vi "Find Average Center_01282025.vi"(5 "Position":i32, 7 "Tray Number":i32, 8 "Assembly Type":string, 9 "XYZTheta":dbl[](array[numeric]), 11 "Gantry In":refnum<k24>) -> (1 "XYZTheta":dbl[](array[numeric]) format="%.6g", 3 "Gantry Out":refnum<k24>)   [LabVIEW 2021, in "Component Tray.lvclass"]
uses:
  Component Tray.lvclass
  Find Component.ctl
  Controller/Camera/Machine Vision.ctl
  C:/Program Files (x86)/Aerotech/A3200/LabVIEW/2010/Bin/Aerotech.A3200.dll
  Program Files (x86)/Aerotech/A3200/LabVIEW/2010/Bin/Aerotech.A3200.dll
  Controller/Camera/Image processing.ctl
  Controller/Camera/Camera settings.ctl
  Controller/Camera/Material.ctl
  Controller/Camera/Edmund Optics/Edmund Optics.lvclass
  C:/Users/User/Documents/Jessica_Code/Jessica_code_08062024/Gantry-CMU/UCSB-Gantry-HEP-main/Classes/Controller/Camera/Camera.lvclass
  Controller/Camera/Camera.lvclass
  Controller/Motion/A3200/A3200.lvclass
  Controller/Motion/Motion.lvclass
  Routine/TypeOfHexaboard.ctl
  Routine/Routine.lvclass
panel:
  out "Low Speed":bool
  out "X":bool
  out "Y":bool
  out "Z":bool
  out "High Speed":bool
  in  "Go to Top Right":bool
  in  "Go to Bottom Right":bool
  out "Program Stopped":bool
  out "XY Graph":cluster{"X":dbl, "Y":dbl}[](graph)
  out "Sensor ID Location":dbl[](array[numeric])
  in  "Go to Sensor ID":bool
  out "CH1 Location":dbl[](array[numeric])
  in  "Verify CH1":bool
  out "CH1 correct?":bool
  in  "Go to CH1":bool
  in  "Focus step size":dbl format="%#_13g"
  in  "number of focus steps":i32
  out "Average Strength":dbl
  in  "Focus":bool
  in  "Material":T1
  out "All fiducials recorded":bool
  in  "Override presets":bool
  in  "Camera settings":T2={"Gamma"=1.6, "Gain"=0, "Sharpness"=0, "Contrast"=0.0, "Exposure"=0.0078125} {"Exposure" min=0.000244140625 max=0.5 scale=0.0002..0.5; "Contrast" min=0.0 max=1.0 scale=0.001..1.0; "Sharpness" min=0 max=2 step=1 scale=0.0..2.0; "Gain" min=0 max=100 step=1 scale=0.1..100.0; "Gamma" min=0.01 max=10.0 scale=0.01..10.0}
  in  "Image processing":T3={"Brightness"=128.0, "Contrast"=45.0, "Gamma"=1.0471123} {"Brightness" scale=0.0..400.0; "Contrast" scale=0.0..90.0; "Gamma" scale=0.005..5.0}
  in  "Machine Vision":T4=enum."Sensor Fiducials"
  out "Gantry":dbl[](array[numeric]) format="%.6g"
  out "Sum":dbl[](array[numeric]) format="%.6g"
  out "Bottom Right XY":dbl[](array[numeric]) format="%.6g"
  out "Bottom Left XY":dbl[](array[numeric]) format="%.6g"
  out "Top Right XY":dbl[](array[numeric]) format="%.6g"
  out "Top Left XY":dbl[](array[numeric]) format="%.6g"
  in  "Record Bottom Left":bool
  in  "Record Bottom Right":bool
  in  "Record Top Right":bool
  in  "Record Top Left":bool
  in  "Go to Bottom Left":bool
  in  "Go to Top Left":bool
  in  "Joystick":bool
  out "Camera":dbl[](array[numeric]) format="%.6g"
  in  "Go to Center":bool
  in  "Component":T5
  in  "Stop Program":bool
  out "Image":T6(plugin-control)
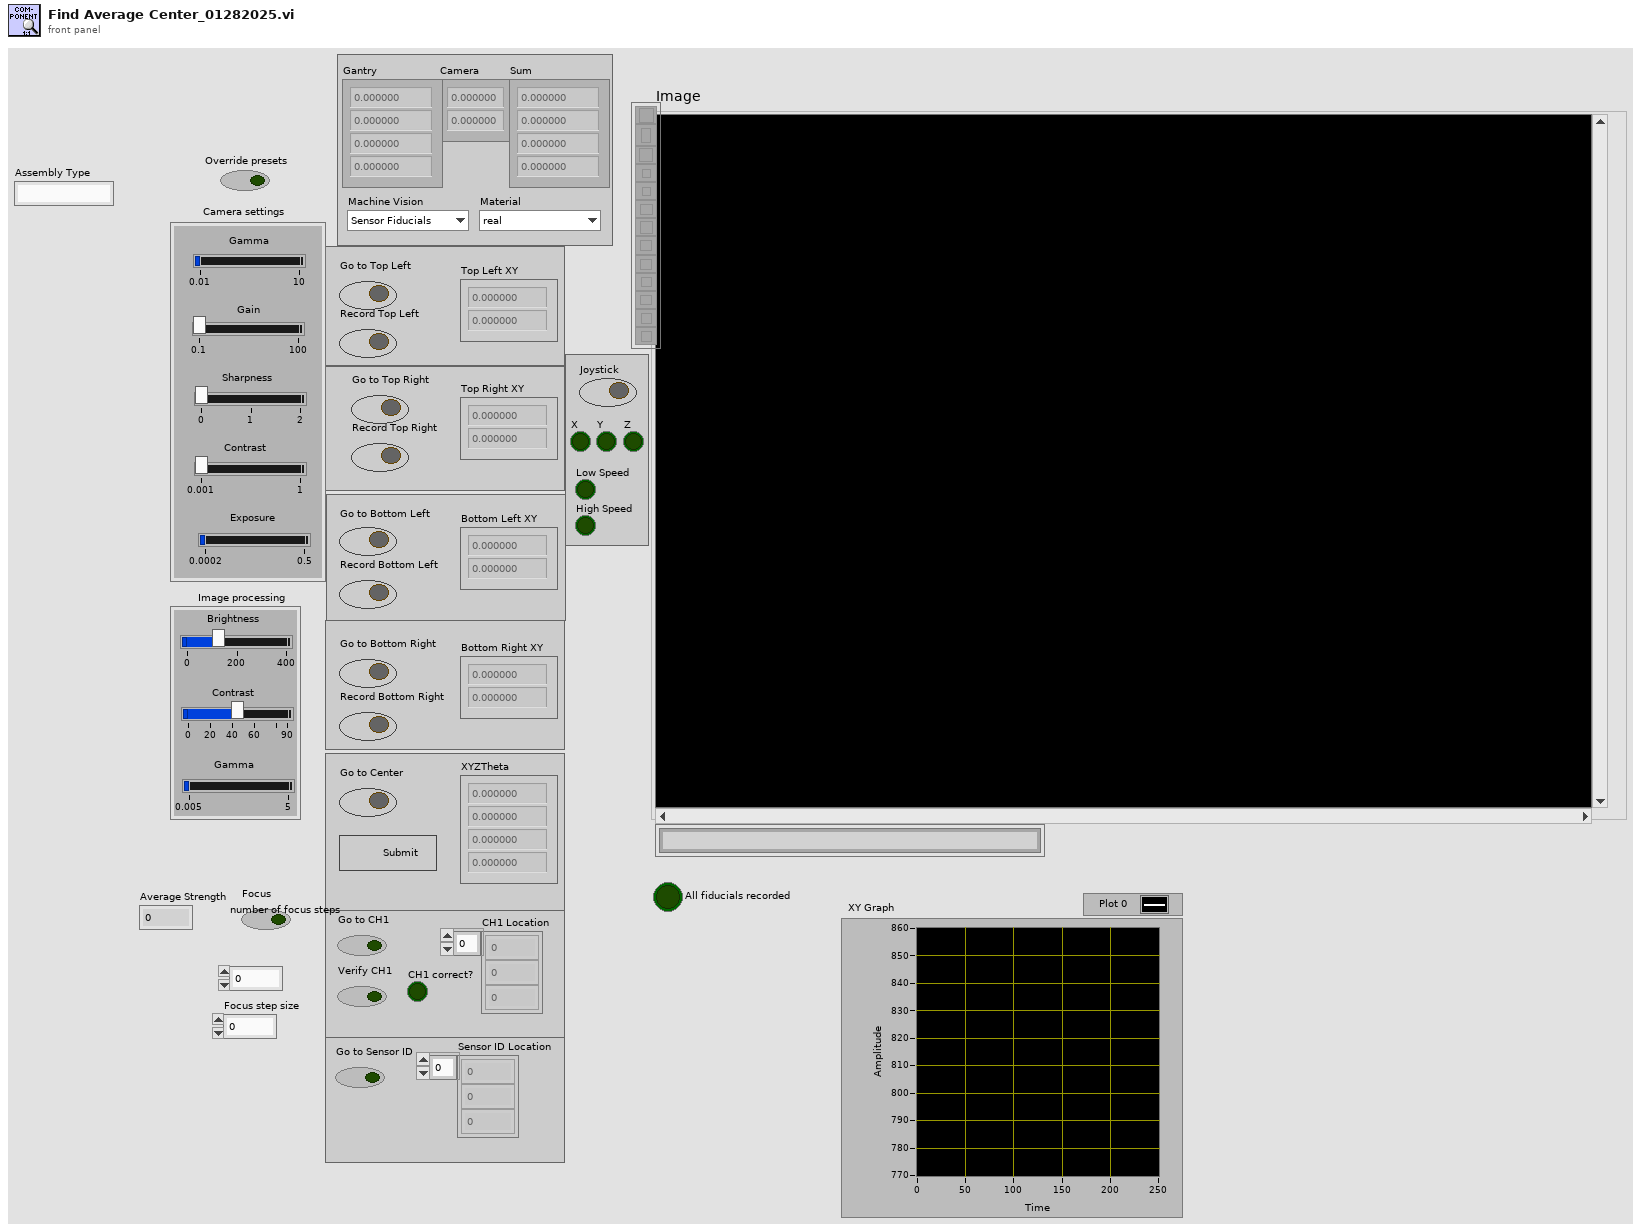
[diagram p1: front panel]
types:
  T1 = typedef "Camera.lvclass/Material.ctl" = enum16{"real", "dummy", "PETG"}
  T2 = typedef "Camera.lvclass/Camera settings.ctl" = cluster{"Gamma":dbl, "Gain":i64, "Sharpness":i64, "Contrast":dbl, "Exposure":dbl}
  T3 = typedef "Camera.lvclass/Image processing.ctl" = cluster{"Brightness":sgl, "Contrast":sgl, "Gamma":sgl}
  T4 = typedef "Camera.lvclass/Machine Vision.ctl" = enum16{"None", "Tray Fiducials", "V3 Sensor Circle", "Partial Hexaboard", "HPK Silicon", "Partial Hexaboard Test", "100um dot", "Hexaboard", "Corner (TL, BR)", "Corner (BL, TR)", "V3 Sensor Cross", "test", "Sensor Fiducials"}
  T5 = typedef "Component Tray.lvclass/Find Component.ctl" = cluster{"New Fiducials":dbl[], "Past Fiducials":dbl[], "XYZTheta":dbl[], "Fiducials Path":path, "Position":i32, "CH1 Location":dbl[], "Sensor ID Location":dbl[]}
  T6 = typedef "IMAQ Image.ctl" = refnum<image>
  T7 = typedef "Routine.lvclass/TypeOfHexaboard.ctl" = enum16{"Full Sensor", "Full PCB", "Right Partial PCB", "Right Partial Sensor", "Al Dummy Right Partial Sensor"}
  T8 = typedef "File Paths.ctl" = cluster{"Glue Pattern Folder":path, "Carrier Tray Folder":path, "Pick Up Tool Fixture Folder":path, "Components Folder":path, "Bellows Tool Offset.txt":path, "Pick Up Tool Offset.txt":path, "Dispense Tip Offset.txt":path, "Log Files":path, "Gantry Assembly Map.txt":path, "Syringe and offset map.txt":path, "Controllers Folder":path, "Local dbase config":path}
  T9 = enum8{"Enabled", "Disabled", "Disabled and Grayed Out"}
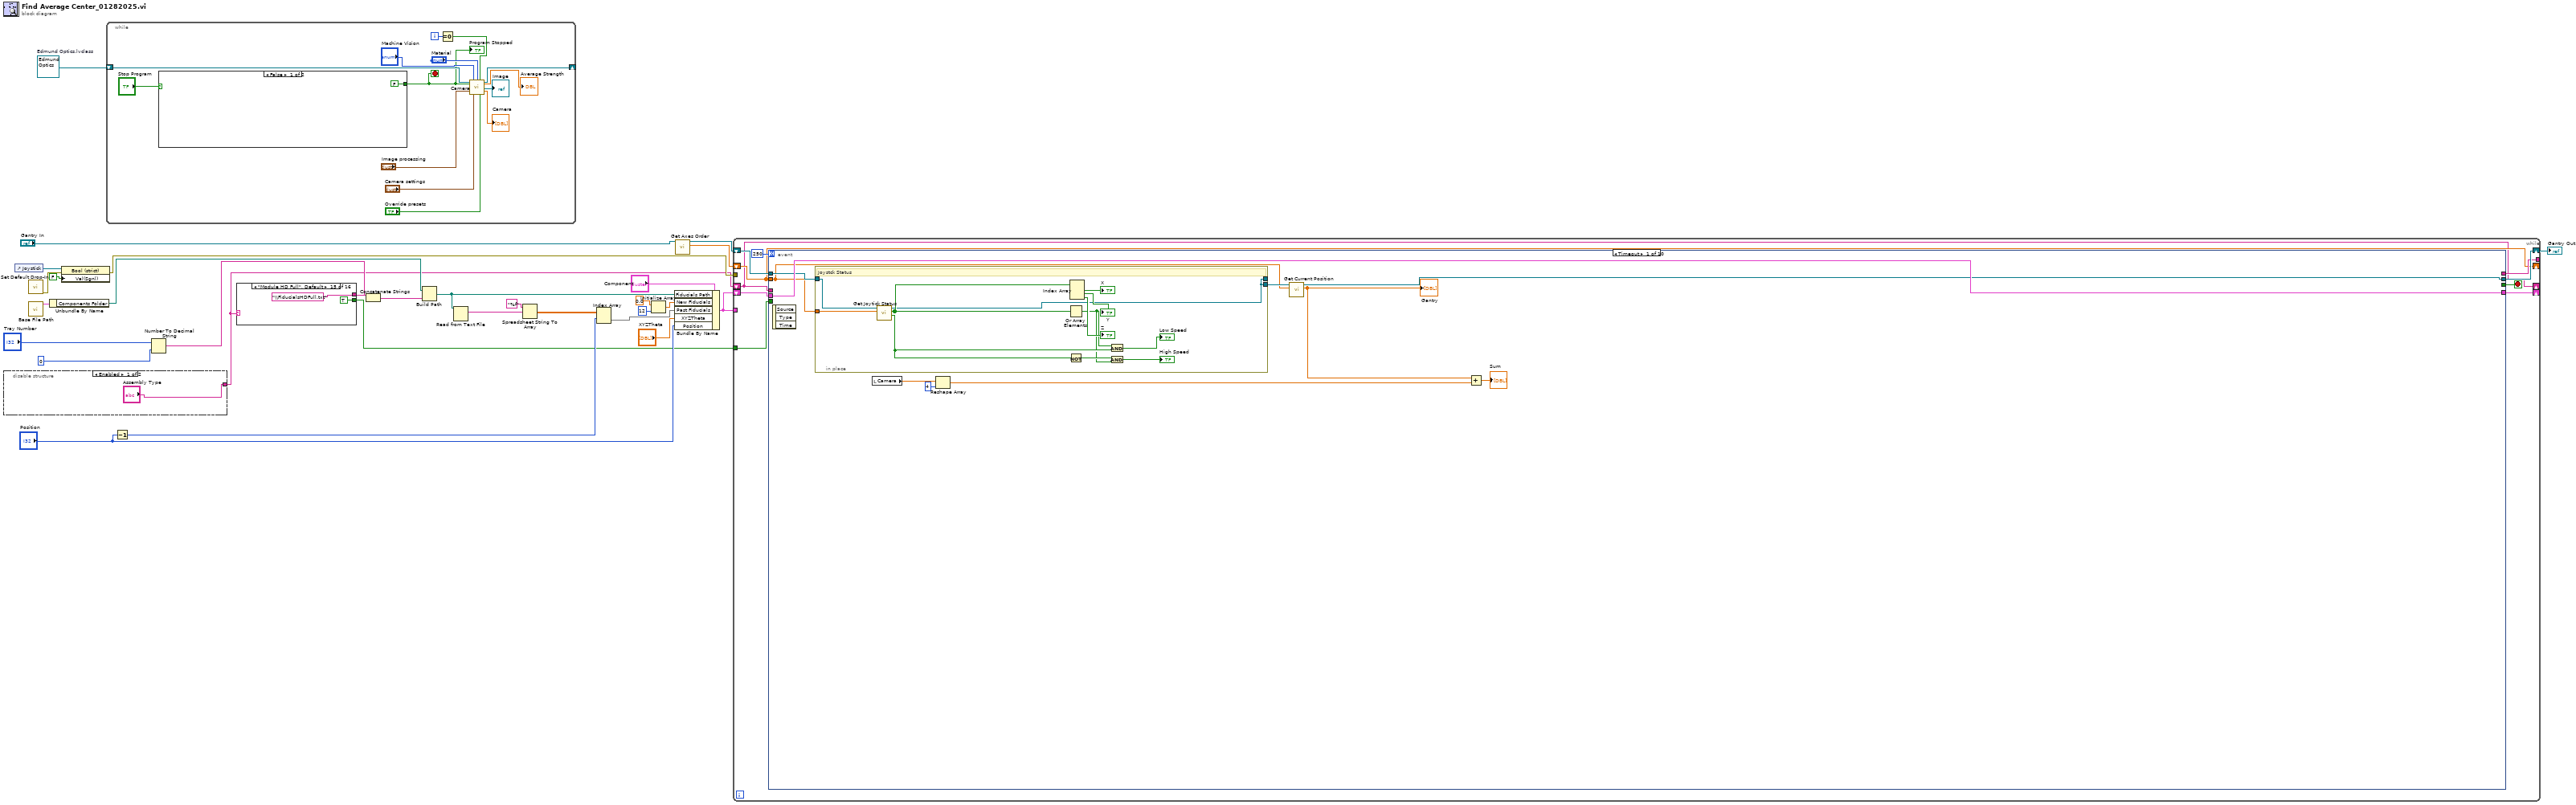
[diagram p0: block diagram]
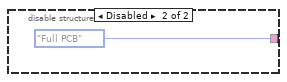
[diagram p2: hidden frame]
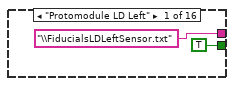
[diagram p3: hidden frame]
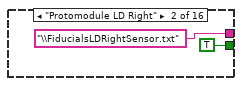
[diagram p4: hidden frame]
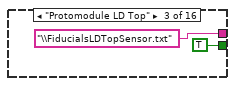
[diagram p5: hidden frame]
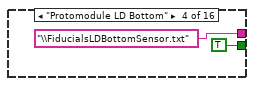
[diagram p6: hidden frame]
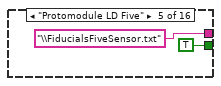
[diagram p7: hidden frame]
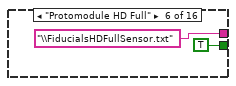
[diagram p8: hidden frame]
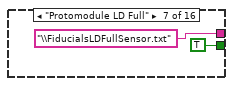
[diagram p9: hidden frame]
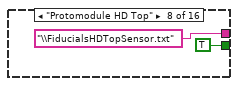
[diagram p10: hidden frame]
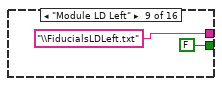
[diagram p11: hidden frame]
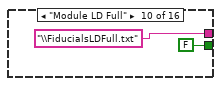
[diagram p12: hidden frame]
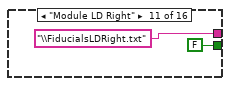
[diagram p13: hidden frame]
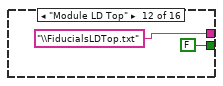
[diagram p14: hidden frame]
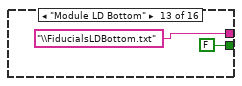
[diagram p15: hidden frame]
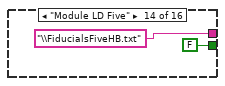
[diagram p16: hidden frame]
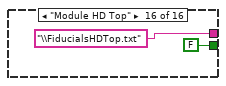
[diagram p17: hidden frame]
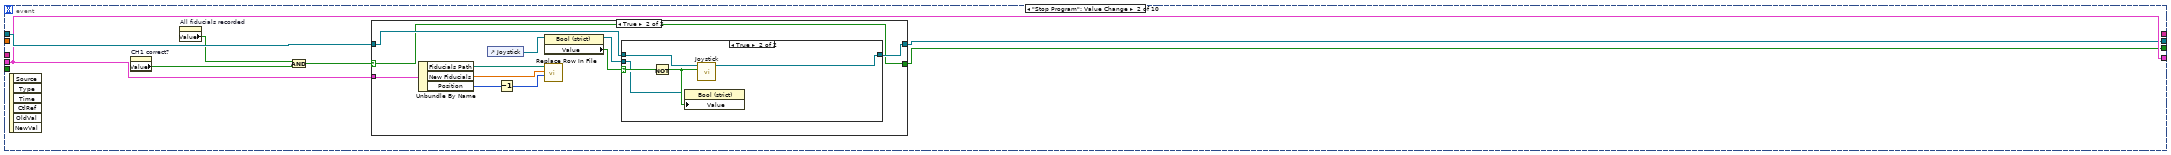
[diagram p18: hidden frame]
diagram:
  w27 = refnum<class "Edmund Optics.lvclass"> refnum  # Edmund Optics.lvclass
  n1 = disable-structure shown="Enabled" {
    disable-tunnel: ["Assembly Type" TypeOfHexaboard."Full PCB" ("Type of Hexaboard")] -> w1
    frame Enabled {
    }
    frame Disabled {
    }
  }
  n2 = control-ref of="Joystick"() -> (w30:refnum<vi>)
  n3 = call "Set Default Drop-In.vi"() -> ("error out"=w8:errorcluster)  [unwired: 11 in]
  n4 = call "Base File Path.vi"() -> ("Paths Out"=w18:T8)  [unwired: 11 in]
  n5 = Unbundle By Name(w18) -> ("Components Folder"=w20:path)
  n6 = property class="Bool (strict)"(reference=w30, error in=w8, "Val(Sgnl)"=FALSE) -> (error out=w28:errorcluster)  [unwired: 1 out]
  n7 = while {
    shift-right: [w43] -> _
    shift-left: w27 -> [w47]
    i -> [w39]
    stop <- w34 stop-if-true
    n8 = case shown="False" "Stop Program" {
      tunnel: [FALSE w49] -> w34
      frame False {
      }
      frame True {
        n9 = property on="All fiducials recorded" class="Bool (strict)"() -> ("Value"=w52:bool)  [unwired: 2 in, 2 out]
        n10 = property on="CH1 correct?" class="Bool (strict)"() -> ("Value"=w50:bool)  [unwired: 2 in, 2 out]
        n11 = And(x=w52, y=w50) -> (x .and. y?=w51:bool)
        n12 = case shown="False" w51 {
          tunnel: [FALSE TRUE] -> w49
          frame False {
            n13 = One Button Dialog(message="At least one fiducial not recorded or component orientation not verified.") -> ()  [unwired: 1 in, 1 out]
          }
          frame True {
            n14 = property on="All fiducials recorded" class="Bool (strict)"("Val(Sgnl)"=FALSE) -> ()  [unwired: 2 in, 2 out]
          }
        }
      }
    }
    "Program Stopped" <- w34
    n15 = Equal To 0?(x=w39) -> (x = 0?=w38:bool)
    n16 = call "Camera.vi"("Camera in"=w47, "Stop"=w34, "BCG Image Processing"="Image processing", "Machine Vision"="Machine Vision", "Camera settings"="Camera settings", "Material"="Material", "Loop 0"=w38, "Override presets"="Override presets") -> ("Camera out"=w43:refnum<class "Edmund Optics.lvclass">, "Average Strength"=→"Average Strength":dbl, "Image"=→"Image":T6, "Camera"=→"Camera":dbl[])  [unwired: 5 in, 3 out]
  }
  n17 = Decrement(x="Position") -> (x-1=w9:i32)
  n18 = Number To Decimal String(number="Tray Number", width (-)=i16 0) -> (decimal integer string=w21:string)
  n19 = case shown="\"Module HD Full\", Default" w1 {
    tunnel: ["\\FiducialsLDLeftSensor.txt" ("string") "\\FiducialsLDRightSensor.txt" ("string") "\\FiducialsLDTopSensor.txt" ("string") "\\FiducialsLDBottomSensor.txt" ("string") "\\FiducialsFiveSensor.txt" ("string") "\\FiducialsHDFullSensor.txt" ("string") "\\FiducialsLDFullSensor.txt" ("string") "\\FiducialsHDTopSensor.txt" ("string") "\\FiducialsLDLeft.txt" ("string") "\\FiducialsLDFull.txt" ("string") "\\FiducialsLDRight.txt" ("string") "\\FiducialsLDTop.txt" ("string") "\\FiducialsLDBottom.txt" ("string") "\\FiducialsFiveHB.txt" ("string") "\\FiducialsHDFull.txt" ("string") "\\FiducialsHDTop.txt" ("string")] -> w22
    tunnel: [TRUE TRUE TRUE TRUE TRUE TRUE TRUE TRUE FALSE FALSE FALSE FALSE FALSE FALSE TRUE FALSE] -> w5
    frame "Protomodule LD Left" {
    }
    frame "Protomodule LD Right" {
    }
    frame "Protomodule LD Top" {
    }
    frame "Protomodule LD Bottom" {
    }
    frame "Protomodule LD Five" {
    }
    frame "Protomodule HD Full" {
    }
    frame "Protomodule LD Full" {
    }
    frame "Protomodule HD Top" {
    }
    frame "Module LD Left" {
    }
    frame "Module LD Full" {
    }
    frame "Module LD Right" {
    }
    frame "Module LD Top" {
    }
    frame "Module LD Bottom" {
    }
    frame "Module LD Five" {
    }
    frame "Module HD Full", Default {
    }
    frame "Module HD Top" {
    }
  }
  n20 = Concatenate Strings "Concatenate Strings"(w21, w22) -> (w23:string)
  n21 = Build Path(base path=w20, name or relative path=w23) -> (appended path=w12:path)
  n22 = Read from Text File(file (use dialog)=w12) -> (text=w24:string)  [unwired: 3 in, 3 out]
  n23 = Spreadsheet String To Array(format string="%f", spreadsheet string=w24) -> (array=w26:dbl[][])  [unwired: 2 in]
  n24 = Index Array "Index Array"(array=w26, index (row)=w9) -> (element=w16:dbl[])  [unwired: 1 in]
  n25 = Initialize Array(0.0 ("element"), 12 ("dimension size")) -> (w15:dbl[])
  n26 = Bundle By Name "Bundle By Name"(cluster="Component", "Fiducials Path"=w12, "New Fiducials"=w15, "Past Fiducials"=w16, "XYZTheta"="XYZTheta", "Position"="Position") -> (w6:T5)
  n27 = call "Get Axes Order.vi"("Gantry In"="Gantry In") -> ("Axes Order"=w2:dbl[], "Gantry Out"=w3:refnum<k24>)  [unwired: 8 in, 1 out]
  n28 = while {
    shift-right: [w96] -> _
    shift-left: w6 -> [w97]
    tunnel: w28 -> [_]
    shift-right: [w93] -> w7
    shift-left: w3 -> [w94]
    tunnel: w6 -> [_]
    tunnel: [w92] -> _
    tunnel: w5 -> [w91]
    shift-right: [w90] -> _
    shift-left: w2 -> [w90]
    shift-right: [w89] -> _
    shift-left: w1 -> [w89]
    stop <- w98 stop-if-true
    n29 = event shown="[0] Timeout" {
      selector: _ -> [_ _ _ _ _ _ _ _ _ _]
      dyn-events: _ -> [_ _ _ _ _ _ _ _ _ _]
      timeout: 250 -> [_ _ _ _ _ _ _ _ _ _]
      tunnel: [_ w124 _ _ _ _ _ _ _ _] -> w98
      tunnel: w97 -> [w107 w126 w163 w227 w366 w414 w421 w436 w451 w461]
      tunnel: [w107 w126 w163 w226 w366 w414 w421 w436 w451 w461] -> w96
      tunnel: w94 -> [w101 w127 w162 w218 w368 w413 w417 w432 w447 w462]
      tunnel: [w103 w125 w159 w216 w367 w411 w415 w430 w445 w462] -> w93
      tunnel: w89 -> [_ _ w156 w215 _ _ _ _ _ _]
      tunnel: [_ _ w156 _ _ _ _ _ _ _] -> w92
      tunnel: w91 -> [_ _ w147 w191 _ _ _ _ _ _]
      tunnel: w90 -> [w99 _ _ w190 w356 _ _ _ _ _]
      event Timeout {
        n30 = event-data() -> ()  [unwired: 1 in, 3 out]
        n31 = in-place {
          in-place-border: w101 -> [w120]
          in-place-border: [w109] -> _
          in-place-border: w99 -> [w119]
          in-place-border: [w109] -> w100
          # "Joystck Status"
          n32 = call "Get Joytick Status.vi"("Axes Order"=w119, "Gantry In"=w120) -> ("JoystickLowSpeedActive"=w113:bool, "Joystick Status"=w115:bool[], "Gantry Out"=w109:refnum<k24>)  [unwired: 6 in, 1 out]
          n33 = Or Array Elements(Boolean array=w115) -> (logical OR=w111:bool)
          n34 = Not(x=w113) -> (.not. x?=w112:bool)
          n35 = Index Array(array=w115) -> (element #1=→"X":bool, element #2=→"Y":bool, element #3=→"Z":bool)  [unwired: 3 in]
          n36 = And(x=w111, y=w113) -> (x .and. y?=→"Low Speed":bool)
          n37 = And(x=w112, y=w111) -> (x .and. y?=→"High Speed":bool)
        }
        n38 = local read "Camera"() -> (w106:dbl[])
        n39 = Reshape Array(w106, 4 ("dimension size")) -> (w104:dbl[])
        n40 = call "Get Current Position.vi"("Axes Order"=w99, "Gantry In"=w100) -> ("XYZTheta Out"=w102:dbl[], "Gantry Out"=w103:refnum<k24>)  [unwired: 7 in, 1 out]
        "Gantry" <- w102
        n41 = Add(x=w102, y=w104) -> (x+y=→"Sum":dbl[])
      }
      event "Stop Program": Value Change {
        n42 = event-data() -> ()  [unwired: 1 in, 6 out]
        n43 = property on="CH1 correct?" class="Bool (strict)"() -> ("Value"=w123:bool)  [unwired: 2 in, 2 out]
        n44 = property on="All fiducials recorded" class="Bool (strict)"() -> ("Value"=w122:bool)  [unwired: 2 in, 2 out]
        n45 = And(x=w122, y=w123) -> (x .and. y?=w121:bool)
        n46 = case shown="True" w121 {
          selector: w121 -> [w128 w137]
          tunnel: w127 -> [w129 w139]
          tunnel: w126 -> [_ w140]
          tunnel: [w129 w138] -> w125
          tunnel: [w128 w137] -> w124
          frame False {
          }
          frame True {
            n47 = Unbundle By Name(w140) -> ("Fiducials Path"=w134:path, "New Fiducials"=w133:dbl[], "Position"=w135:i32)
            n48 = control-ref of="Joystick"() -> (w131:refnum<vi>)
            n49 = Decrement(x=w135) -> (x-1=w136:i32)
            n50 = property class="Bool (strict)"(reference=w131) -> (reference out=w130:refnum<vi>, "Value"=w132:bool)  [unwired: 1 in, 1 out]
            n51 = call "Replace Row In File.vi"("Index"=w136, "Insert Array"=w133, "Path"=w134) -> ()  [unwired: 8 in, 1 out]
            n52 = case shown="True" w132 {
              selector: w132 -> [_ w146]
              tunnel: w139 -> [w141 w145]
              tunnel: [w141 w144] -> w138
              tunnel: w130 -> [_ w142]
              frame False {
              }
              frame True {
                n53 = Not(x=w146) -> (.not. x?=w143:bool)
                n54 = property class="Bool (strict)"(reference=w142, "Value"=w143) -> ()  [unwired: 1 in, 2 out]
                n55 = call "Joystick.vi"("Joystick"=w143, "Gantry In"=w145) -> ("Gantry Out"=w144:refnum<k24>)  [unwired: 8 in, 1 out]
              }
            }
          }
        }
      }
      event "Go to Top Left", "Go to Bottom Left", "Go to Bottom Right", "Go to Top Right": Value Change {
        n56 = event-data() -> ()  [unwired: 1 in, 6 out]
        n57 = disable-structure shown="Enabled" {
          disable-tunnel: w162 -> [w169 _]
          disable-tunnel: [w168 _] -> w161
          frame Enabled {
            n58 = control-ref of="Joystick"() -> (w167:refnum<vi>)
            n59 = property class="Bool (strict)"(reference=w167) -> (reference out=w170:refnum<vi>, "Value"=w171:bool)  [unwired: 1 in, 1 out]
            n60 = case shown="True" w171 {
              selector: w171 -> [_ w177]
              tunnel: w169 -> [w172 w175]
              tunnel: [w172 w173] -> w168
              tunnel: w170 -> [_ w176]
              frame False {
              }
              frame True {
                n61 = Not(x=w177) -> (.not. x?=w174:bool)
                n62 = call "Joystick.vi"("Joystick"=w174, "Gantry In"=w175) -> ("Gantry Out"=w173:refnum<k24>)  [unwired: 8 in, 1 out]
                n63 = property class="Bool (strict)"(reference=w176, "Value"=w174) -> ()  [unwired: 1 in, 2 out]
              }
            }
          }
          frame Disabled {
          }
        }
        n64 = Unbundle By Name(w163) -> ("Past Fiducials"=w165:dbl[])
        n65 = Build Array "Build Array"("Go to Top Left", "Go to Top Right", "Go to Bottom Left", "Go to Bottom Right") -> (w166:bool[])
        n66 = Select(t=T9."Enabled" ("Disabled"), s=w147, f=T9."Disabled and Grayed Out" ("Disabled")) -> (s? t:f=w148:T9)
        n67 = Select(t=T9."Enabled" ("Disabled"), s=w147, f=T9."Disabled and Grayed Out" ("Disabled")) -> (s? t:f=w151:T9)
        n68 = for {
          tunnel: w166 -> [w189] mode=indexing
          tunnel: w165 -> [w188]
          tunnel: [w183] -> w164 if=w189
          i -> [w186]
          n69 = Multiply(x=w186, y=3) -> (x*y=w184:i32)
          n70 = Array Subset "Array Subset"(array=w188, index=w184, length=3) -> (w183:dbl[])
        }
        n71 = property on="Go to Bottom Right" class="Bool"("DisabledEnum"=w148) -> ()  [unwired: 2 in, 2 out]
        n72 = property on="Go to Top Right" class="Bool"("DisabledEnum"=w151) -> ()  [unwired: 2 in, 2 out]
        n73 = call "ClearXYZTheta Go.vi"("XYZTheta In"=w164, "Gantry In"=w161) -> ("Gantry Out"=w160:refnum<k24>)  [unwired: 7 in, 2 out]
        n74 = flat-sequence {
          tunnel: w160 -> [w182]
          tunnel: [w179] -> w159
          frame #0 {
            w178 = TRUE
            n75 = control-ref of="Joystick"() -> (w181:refnum<vi>)
            n76 = call "Joystick.vi"("Joystick"=w178, "Gantry In"=w182) -> ("error out"=w180:errorcluster, "Gantry Out"=w179:refnum<k24>)  [unwired: 8 in]
            n77 = property on="Property Node" class="Bool (strict)"(reference=w181, error in=w180, "Value"=w178) -> ()  [unwired: 2 out]
          }
        }
      }
      event "Record Top Left", "Record Top Right", "Record Bottom Right", "Record Bottom Left": Value Change {
        n78 = event-data() -> ()  [unwired: 1 in, 1 out]
        n79 = call "Get Current Position.vi"("Axes Order"=w190, "Gantry In"=w218) -> ("XYZTheta Out"=w217:dbl[], "Gantry Out"=w216:refnum<k24>)  [unwired: 7 in, 1 out]
        n80 = control-ref of="Top Left XY"() -> (w213:refnum<vi>)
        n81 = control-ref of="Bottom Left XY"() -> (w211:refnum<vi>)
        n82 = local read "Camera"() -> (w221:dbl[])
        n83 = control-ref of="Bottom Right XY"() -> (w210:refnum<vi>)
        n84 = control-ref of="Top Right XY"() -> (w212:refnum<vi>)
        n85 = Reshape Array(w221, 3 ("dimension size")) -> (w220:dbl[])
        n86 = Build Array "Build Array"(w213, w212, w211, w210) -> (w225:refnum<vi>[])
        n87 = Add(x=w217, y=w220) -> (x+y=w219:dbl[])
        n88 = Select(t=T9."Enabled" ("Disabled"), s=w191, f=T9."Disabled and Grayed Out" ("Disabled")) -> (s? t:f=w192:T9)
        n89 = Select(t=T9."Enabled" ("Disabled"), s=w191, f=T9."Disabled and Grayed Out") -> (s? t:f=w202:T9)
        n90 = Select(t=T9."Enabled" ("Disabled"), s=w191, f=T9."Disabled and Grayed Out" ("Disabled")) -> (s? t:f=w196:T9)
        n91 = Select(t=T9."Enabled" ("Disabled"), s=w191, f=T9."Disabled and Grayed Out") -> (s? t:f=w200:T9)
        n92 = Build Array "Build Array"("Record Top Left", "Record Top Right", "Record Bottom Left", "Record Bottom Right") -> (w214:bool[])
        n93 = for {
          tunnel: w214 -> [w228] mode=indexing
          tunnel: [w229] -> w205 if=w228
          i -> [w229]
        }
        n94 = property on="Record Top Right" class="Bool"("DisabledEnum"=w202) -> ()  [unwired: 2 in, 2 out]
        n95 = property on="Top Right XY" class="Arr (strict)"("DisabledEnum"=w196) -> ()  [unwired: 2 in, 2 out]
        n96 = property on="Record Bottom Right" class="Bool"("DisabledEnum"=w200) -> ()  [unwired: 2 in, 2 out]
        n97 = property on="Bottom Right XY" class="Arr (strict)"("DisabledEnum"=w192) -> ()  [unwired: 2 in, 2 out]
        n98 = Index Array "Index Array"(array=w225, index=w205) -> (element=w224:refnum<vi>)
        n99 = Multiply(x=w205, y=3) -> (x*y=w222:i32)
        n100 = in-place {
          in-place-border: w222 -> [w233]
          in-place-border: w224 -> [w251]
          in-place-border: w219 -> [w234]
          in-place-border: w215 -> [w238]
          in-place-border: w191 -> [w236]
          n101 = in-place-cluster #1(w227) -> ("New Fiducials"=w235:dbl[], "XYZTheta"=w250:dbl[], "Position"=w231:i32)  [unwired: 2 out]
          n102 = case shown="False" w236 {
            tunnel: w235 -> [w259 _]
            tunnel: w233 -> [w258 _]
            tunnel: w234 -> [w257 _]
            tunnel: [w254 w260] -> w237
            tunnel: w235 -> [_ w263]
            tunnel: w234 -> [_ w262]
            tunnel: w233 -> [_ w261]
            tunnel: [w254 w260] -> w232
            frame False {
              n103 = Add(x=w258, y=3) -> (x+y=w255:i32)
              n104 = Replace Array Subset "Replace Array Subset"(array=w259, new element #1=w257, index #1=w258, new element #2=w257, index #2=w255) -> (w254:dbl[])
            }
            frame True {
              n105 = Replace Array Subset "Replace Array Subset"(array=w263, new element=w262, index=w261) -> (w260:dbl[])
            }
          }
          n106 = property class="Arr (strict)"(reference=w251, "Value"=w234) -> ()  [unwired: 1 in, 2 out]
          n107 = Array Subset "Array Subset"(array=w232, length=12) -> (w245:dbl[])  [unwired: 1 in]
          n108 = Multiply Array Elements(1:w245) -> (0:w248:dbl)
          n109 = Reshape Array "Reshape Array"(w245, 4 ("dimension size"), 3 ("dimension size")) -> (w242:dbl[][])
          n110 = for {
            tunnel: w242 -> [w264] mode=indexing
            tunnel: [w265] -> w241 mode=indexing
            n111 = Index Array(array=w264) -> ()  [unwired: 2 in, 2 out]
            n112 = Array To Cluster(array=w264) -> (cluster=w265:cluster{"[0]":dbl, "[1]":dbl})
          }
          n113 = Not Equal To 0?(x=w248) -> (x != 0?=w239:bool)
          "All fiducials recorded" <- w239
          n114 = case shown="True" w239 {
            tunnel: [w269 w276] -> w253
            tunnel: w237 -> [w270 w280]
            tunnel: [w270 w280] -> w252
            tunnel: w250 -> [w269 _]
            tunnel: [w268 w277] -> w247
            tunnel: [w268 w278] -> w246
            tunnel: w241 -> [w267 w283]
            tunnel: [w267 w281] -> w240
            tunnel: w238 -> [_ w279]
            tunnel: w231 -> [w266 w274]
            tunnel: [w266 w273] -> w230
            frame False {
              w268 = dbl[] [] ("CH1 location")
            }
            frame True {
              n115 = case shown="\"Protomodule LD Left\"" w279 {
                tunnel: ["calculate_center" ("function name") "calculate_center_adjY_axisY" ("function name") "calculate_center_adjY_axisY" ("function name") "calculate_center_adjX_axisY" ("function name") "calculate_center_adjX_axisY" ("function name") "calculate_center" ("function name") "calculate_center" ("function name") "calculate_center_adjX_axisY" ("function name") "calculate_center" ("function name") "calculate_center_adjY_axisX" ("function name") "calculate_center_adjY_axisX" ("function name") "calculate_center_adjX_axisY" ("function name") "calculate_center_adjX_axisY" ("function name") "calculate_center_adjY_axisX" ("function name") "calculate_center" ("function name") "calculate_center_adjX_axisY" ("function name")] -> w275
                tunnel: [0.0 -45.14 45.14 41.64 -41.64 0.0 0.0 49.78 0.0 -2.0 28.0 2.0 -1.38 0.0 0.0 21.0] -> w272
                tunnel: [1 0 1 1 1 1 1 1 1 0 1 1 1 1 1 1] -> w271
                frame "Protomodule LD Full", Default {
                }
                frame "Protomodule LD Left" {
                }
                frame "Protomodule LD Right" {
                }
                frame "Protomodule LD Top" {
                }
                frame "Protomodule LD Bottom" {
                }
                frame "Protomodule LD Five" {
                }
                frame "Protomodule HD Full" {
                }
                frame "Protomodule HD Top" {
                }
                frame "Module LD Full" {
                }
                frame "Module LD Left" {
                }
                frame "Module LD Right" {
                }
                frame "Module LD Top" {
                }
                frame "Module LD Bottom" {
                }
                frame "Module LD Five" {
                }
                frame "Module HD Full" {
                }
                frame "Module HD Top" {
                }
              }
              n116 = Index Array(array=w283) -> (element=w282:cluster{"[0]":dbl, "[1]":dbl})  [unwired: 1 in]
              n117 = Build Array (concatenate)(w283, w282) -> (w281:cluster{"[0]":dbl, "[1]":dbl}[])
              n118 = disable-structure shown="Enabled" {
                disable-tunnel: w280 -> [w294 w304]
                disable-tunnel: [w290 w307] -> w278
                disable-tunnel: [w291 w306] -> w277
                disable-tunnel: [w292 w305] -> w276
                disable-tunnel: w275 -> [w289 _]
                disable-tunnel: w274 -> [w286 _]
                disable-tunnel: [w286 _] -> w273
                disable-tunnel: w272 -> [w285 _]
                disable-tunnel: w271 -> [w284 _]
                frame Enabled {
                  n119 = call "Base File Path.vi"() -> ("Paths Out"=w299:T8)  [unwired: 11 in]
                  n120 = Unbundle By Name(w299) -> ("Components Folder"=w297:path)
                  n121 = call "Get Python Version.vi"() -> ("Python Version"=w288:string, "error out"=w287:errorcluster)  [unwired: 10 in]
                  n122 = Open Python Session(python version=w288, 3:w287) -> (session out=w303:refnum<k35>, error out=w301:errorcluster)  [unwired: 1 in]
                  n123 = Build Path(base path=w297, name or relative path=path "Calculate Component Center.py") -> (appended path=w296:path)
                  n124 = node(w303, w296, w289, w301, dbl[][] [], w294, w286, w285, w284) -> (w302:refnum<k35>, w300:errorcluster, w293:dbl[][])  [unwired: 4 in, 2 out]
                  n125 = Close Python Session(session in=w302, error in=w300) -> ()  [unwired: 1 out]
                  n126 = Index Array(array=w293) -> (element #1=w292:dbl[], element #2=w291:dbl[], element #3=w290:dbl[])  [unwired: 6 in]
                }
                frame Disabled {
                  n127 = call "Calculate Average Center.vi"("Gantry Fiducials"=w304) -> ("Sensor ID Location"=w307:dbl[], "CH1 Location"=w306:dbl[], "XYZTheta"=w305:dbl[])  [unwired: 8 in]
                }
              }
              "XYZTheta" <- w276
            }
          }
          "CH1 Location" <- w247
          "Sensor ID Location" <- w246
          "XY Graph" <- w240
          n128 = in-place-cluster #1("New Fiducials"=w252, "XYZTheta"=w253, "CH1 Location"=w247, "Sensor ID Location"=w246, "Position"=w230) -> (w226:T5)
        }
      }
      event "Focus": Value Change {
        n129 = event-data() -> ()  [unwired: 1 in, 6 out]
        n130 = Divide(x="number of focus steps", y=2) -> (x/y=w371:dbl)
        n131 = Multiply(x=w371, y="Focus step size") -> (x*y=w369:dbl)
        n132 = call "Joystick.vi"("Joystick"=FALSE, "Gantry In"=w368) -> ("Gantry Out"=w362:refnum<k24>)  [unwired: 8 in, 1 out]
        n133 = Negate(x=w369) -> (-x=w363:dbl)
        n134 = call "Z Go.vi"("Increment"=TRUE, "Return Immediately"=FALSE ("Increment"), "Speed In"=1.0 ("Speed"), "Position In"=w363, "Gantry In"=w362) -> ("error out"=w360:errorcluster, "Gantry Out"=w361:refnum<k24>)  [unwired: 3 in, 2 out]
        n135 = for {
          N: "number of focus steps" -> [_]
          tunnel: [w389] -> w382 mode=indexing
          tunnel: w360 -> [w388]
          tunnel: [w386] -> w375
          shift-right: [w390] -> w376
          shift-left: w361 -> [w392]
          tunnel: "Focus step size" -> [w385]
          tunnel: w356 -> [w384]
          n136 = flat-sequence {
            tunnel: w392 -> [w400]
            tunnel: [w399] -> w391
            tunnel: w388 -> [w398]
            tunnel: [w397] -> w387
            tunnel: w385 -> [w395]
            tunnel: w391 -> [w410]
            tunnel: [w409] -> w390
            tunnel: [w408] -> w389
            tunnel: w387 -> [w404]
            tunnel: [w403] -> w386
            tunnel: w384 -> [w401]
            frame #0 {
              n137 = call "Z Go.vi"("Increment"=TRUE, "Return Immediately"=FALSE ("Increment"), "error in (no error)"=w398, "Speed In"=0.1 ("Speed"), "Position In"=w395, "Gantry In"=w400) -> ("error out"=w397:errorcluster, "Gantry Out"=w399:refnum<k24>)  [unwired: 2 in, 2 out]
            }
            frame #1 {
              n138 = call "Get Current Position.vi"("error in (no error)"=w404, "Axes Order"=w401, "Gantry In"=w410) -> ("error out"=w403:errorcluster, "XYZTheta Out"=w407:dbl[], "Gantry Out"=w409:refnum<k24>)  [unwired: 6 in]
              n139 = local read "Average Strength"() -> (w402:dbl)
              n140 = Delete From Array(array=w407, index=2) -> (deleted portion=w405:dbl)  [unwired: 1 in, 1 out]
              n141 = Build Array(w402, w405) -> (w408:dbl[])
            }
          }
        }
        n142 = Transpose 2D Array(2D array=w382) -> (transposed array=w381:dbl[][])
        n143 = Index Array(array=w381) -> (element #2=w380:dbl[])  [unwired: 4 in, 1 out]
        n144 = Index Array(array=w381) -> (element=w383:dbl[])  [unwired: 2 in]
        n145 = Array Max & Min(array=w383) -> (max index (indices)=w379:i32)  [unwired: 3 out]
        n146 = Index Array(array=w380, index=w379) -> (element=w378:dbl)
        n147 = call "Z Go.vi"("Increment"=FALSE, "Return Immediately"=FALSE ("Increment"), "error in (no error)"=w375, "Speed In"=15.0 ("Speed"), "Position In"=w378, "Gantry In"=w376) -> ("Gantry Out"=w367:refnum<k24>)  [unwired: 2 in, 3 out]
      }
      event "Joystick": Value Change {
        n148 = event-data() -> ()  [unwired: 1 in, 6 out]
        n149 = call "Joystick.vi"("Joystick"="Joystick", "Gantry In"=w413) -> ("Gantry Out"=w411:refnum<k24>)  [unwired: 8 in, 1 out]
      }
      event "Go to Center": Value Change {
        n150 = event-data() -> ()  [unwired: 1 in, 6 out]
        n151 = Unbundle By Name(w421) -> ("XYZTheta"=w422:dbl[])
        n152 = control-ref of="Joystick"() -> (w418:refnum<vi>)
        n153 = property class="Bool (strict)"(reference=w418) -> (reference out=w419:refnum<vi>, "Value"=w420:bool)  [unwired: 1 in, 1 out]
        n154 = case shown="True" w420 {
          selector: w420 -> [_ w429]
          tunnel: w417 -> [w423 w426]
          tunnel: [w423 w425] -> w416
          tunnel: w419 -> [_ w428]
          frame False {
          }
          frame True {
            n155 = Not(x=w429) -> (.not. x?=w424:bool)
            n156 = call "Joystick.vi"("Joystick"=w424, "Gantry In"=w426) -> ("error out"=w427:errorcluster, "Gantry Out"=w425:refnum<k24>)  [unwired: 8 in]
            n157 = property class="Bool (strict)"(reference=w428, error in=w427, "Value"=w424) -> ()  [unwired: 2 out]
          }
        }
        n158 = call "ClearXYZTheta Go.vi"("XYZTheta In"=w422, "Gantry In"=w416) -> ("Gantry Out"=w415:refnum<k24>)  [unwired: 7 in, 2 out]
      }
      event "Go to CH1": Value Change {
        n159 = event-data() -> ()  [unwired: 1 in, 6 out]
        n160 = Unbundle By Name(w436) -> ("CH1 Location"=w437:dbl[])
        n161 = control-ref of="Joystick"() -> (w433:refnum<vi>)
        n162 = property class="Bool (strict)"(reference=w433) -> (reference out=w434:refnum<vi>, "Value"=w435:bool)  [unwired: 1 in, 1 out]
        n163 = case shown="True" w435 {
          selector: w435 -> [_ w444]
          tunnel: w432 -> [w438 w441]
          tunnel: [w438 w440] -> w431
          tunnel: w434 -> [_ w443]
          frame False {
          }
          frame True {
            n164 = Not(x=w444) -> (.not. x?=w439:bool)
            n165 = call "Joystick.vi"("Joystick"=w439, "Gantry In"=w441) -> ("error out"=w442:errorcluster, "Gantry Out"=w440:refnum<k24>)  [unwired: 8 in]
            n166 = property class="Bool (strict)"(reference=w443, error in=w442, "Value"=w439) -> ()  [unwired: 2 out]
          }
        }
        n167 = call "ClearXYZTheta Go.vi"("XYZTheta In"=w437, "Gantry In"=w431) -> ("Gantry Out"=w430:refnum<k24>)  [unwired: 7 in, 2 out]
      }
      event "Go to Sensor ID": Value Change {
        n168 = event-data() -> ()  [unwired: 1 in, 6 out]
        n169 = Unbundle By Name(w451) -> ("Sensor ID Location"=w452:dbl[])
        n170 = control-ref of="Joystick"() -> (w448:refnum<vi>)
        n171 = property class="Bool (strict)"(reference=w448) -> (reference out=w449:refnum<vi>, "Value"=w450:bool)  [unwired: 1 in, 1 out]
        n172 = case shown="True" w450 {
          selector: w450 -> [_ w459]
          tunnel: w447 -> [w453 w456]
          tunnel: [w453 w455] -> w446
          tunnel: w449 -> [_ w458]
          frame False {
          }
          frame True {
            n173 = Not(x=w459) -> (.not. x?=w454:bool)
            n174 = call "Joystick.vi"("Joystick"=w454, "Gantry In"=w456) -> ("error out"=w457:errorcluster, "Gantry Out"=w455:refnum<k24>)  [unwired: 8 in]
            n175 = property class="Bool (strict)"(reference=w458, error in=w457, "Value"=w454) -> ()  [unwired: 2 out]
          }
        }
        n176 = call "ClearXYZTheta Go.vi"("XYZTheta In"=w452, "Gantry In"=w446) -> ("Gantry Out"=w445:refnum<k24>)  [unwired: 7 in, 2 out]
      }
      event "Verify CH1": Value Change {
        n177 = event-data() -> ()  [unwired: 1 in, 6 out]
        "CH1 correct?" <- TRUE
      }
    }
  }
  "Gantry Out" <- w7
